vi "簇和数组.vi"() -> ()   [LabVIEW 2018]
panel:
  out "波形图 4":cluster{dbl, dbl, dbl[][]}(graph)
  out "波形图 3":cluster{dbl, dbl, dbl[]}[](graph)
  out "波形图 2":cluster{dbl[]}[](graph)
  out "波形图":dbl[][](graph)
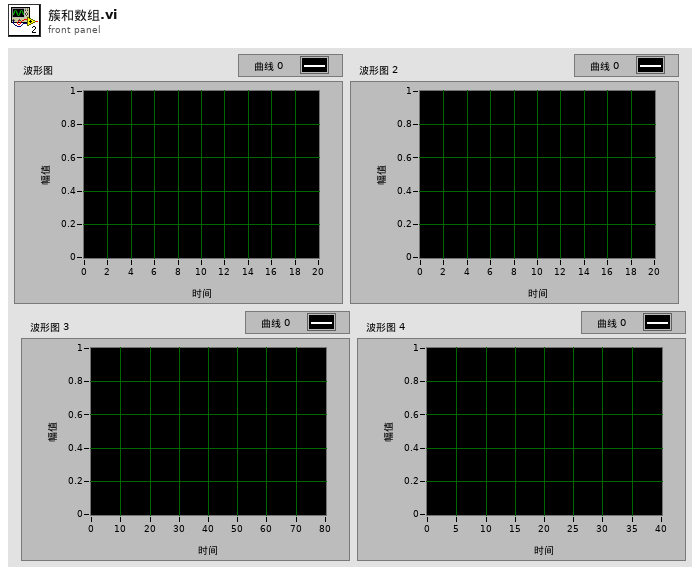
[diagram p1: front panel]
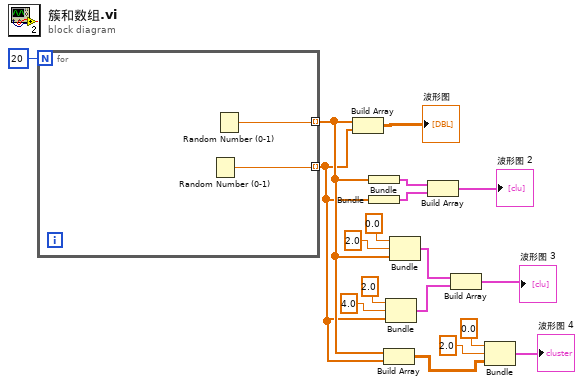
[diagram p0: block diagram]
diagram:
  n1 = for {
    N: 20 -> [_]
    tunnel: [w20] -> w5 mode=indexing
    tunnel: [w19] -> w4 mode=indexing
    n2 = Random Number (0-1)() -> (number: 0 to 1=w19:dbl)
    n3 = Random Number (0-1)() -> (number: 0 to 1=w20:dbl)
  }
  n4 = Build Array(w5, w4) -> (→"波形图":dbl[][])
  n5 = Bundle(w5) -> (w18:cluster{dbl[]})  [unwired: 1 in]
  n6 = Bundle(w4) -> (w17:cluster{dbl[]})  [unwired: 1 in]
  n7 = Build Array(w5, w4) -> (w3:dbl[][])
  n8 = Bundle(2.0, 4.0, w4) -> (w9:cluster{dbl, dbl, dbl[]})  [unwired: 1 in]
  n9 = Bundle(0.0, 2.0, w5) -> (w10:cluster{dbl, dbl, dbl[]})  [unwired: 1 in]
  n10 = Build Array(w18, w17) -> (→"波形图 2":cluster{dbl[]}[])
  n11 = Build Array(w10, w9) -> (→"波形图 3":cluster{dbl, dbl, dbl[]}[])
  n12 = Bundle(0.0, 2.0, w3) -> (→"波形图 4":cluster{dbl, dbl, dbl[][]})  [unwired: 1 in]
